vi "VisualizeRoomAlert.vi"() -> ()   [LabVIEW 2018, in "Visualization.lvlib" / "VisualizeSensor.lvclass"]
doc: "This VI listens for any measurement data associated with the provided PluginName and displays it to the user for analysis. The display is only suitable for data coming from the RoomAlert Plugin."
uses:
  VisualizeSensor.lvclass
  VisualizeBase/VisualizeBase_class/Requests/clUserEventType.ctl
  <vilib>/event_ctls.llb/usereventprio.ctl
  Sensor/SensorShared/clSensorData.ctl
  <vilib>/Utility/error.llb/Error Cluster From Error Code.vi
  <vilib>/ErrorRing/Error Ring.xnode
  <userlib>/NIST/NISTErrorLib/NISTErrorLib.lvlib
  VisualizeBase/VisualizeBase_class/VisualizeBase.lvclass
  Sensor/SensorShared/SensorShared.lvlib
  Sensor/SensorModule/SensorModule.lvlib
panel:
  out "LightTower":T1(array[cluster])
  out "String Results":string[](array[string])
  in  "Tab Control":enum32{"Chart"}(tab)
  out "Siemens":waveform(dbl)[](graph)=[{"t0"=timestamp(3657200531.6397257 s since 1904-01-01), "dt"=1.0, "Y"=[46.19]}, {"t0"=timestamp(3657200531.6397257 s since 1904-01-01), "dt"=1.0, "Y"=[2.0]}, {"t0"=timestamp(3657200531.6397257 s since 1904-01-01), "dt"=1.0, "Y"=[60.0]}]
  in  "PlotYAxis":u32[](array[numeric])=[0, 1, 0] max=1
  out "Incorrect DataType?":bool
  out "ErrorArray":errorcluster[](array[cluster])
  in  "PluginName":string="Sensor.RoomAlert0"
  in  "btnStop":bool
  in  "btnReset":bool
  in  "btnClear":bool
  # "0=Left Axis and 1=Right Axis"
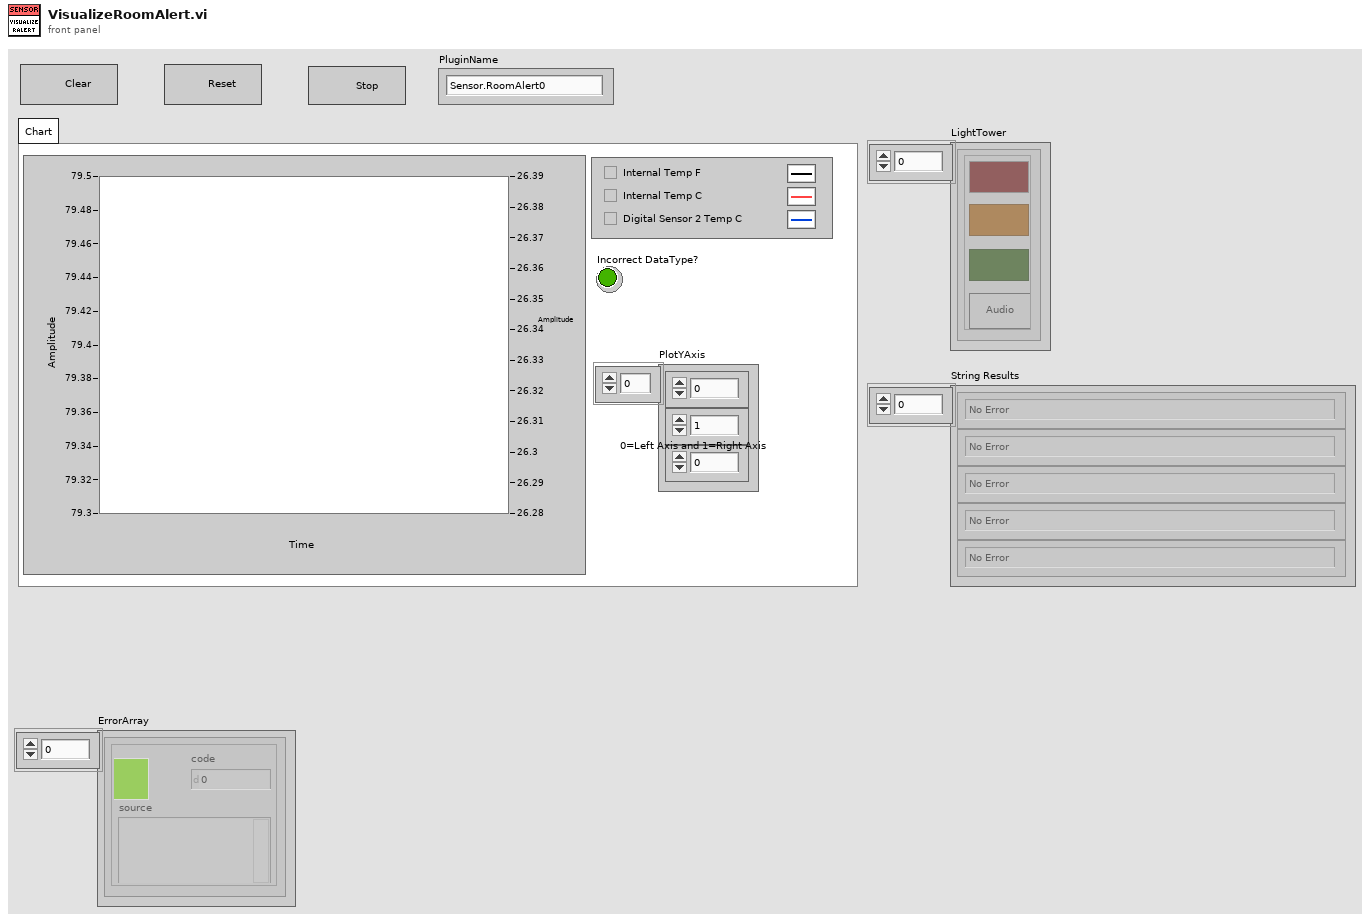
[diagram p1: front panel]
types:
  T1 = cluster{"Red":bool, "Amber":bool, "Green":bool, "Audio":bool}[]
  T2 = typedef "Visualization.lvlib/VisualizeBase.lvclass/clRequestEvents.ctl" = cluster{"StopRequest":refnum<user-event>, "ResetRequest":refnum<user-event>}
  T3 = typedef "SensorShared.lvlib/clBroadcastEvents.ctl" = cluster{"DidInit":refnum<user-event>, "StatusUpdate":refnum<user-event>, "ErrorReport":refnum<user-event>, "DidStop":refnum<user-event>, "PathToINI":refnum<user-event>, "SensorReport":refnum<user-event>, "SensorConfig":refnum<user-event>}
  T4 = typedef "SensorShared.lvlib/clSensorData.ctl" = cluster{"SensorType":string, "SensorData":variant}
  T5 = typedef "Visualization.lvlib/VisualizeBase.lvclass/clUserEventType.ctl" = cluster{"BusIndex":i8, "Data":variant}
  T6 = typedef "usereventprio.ctl" = enum32{"high priority", "normal priority"}
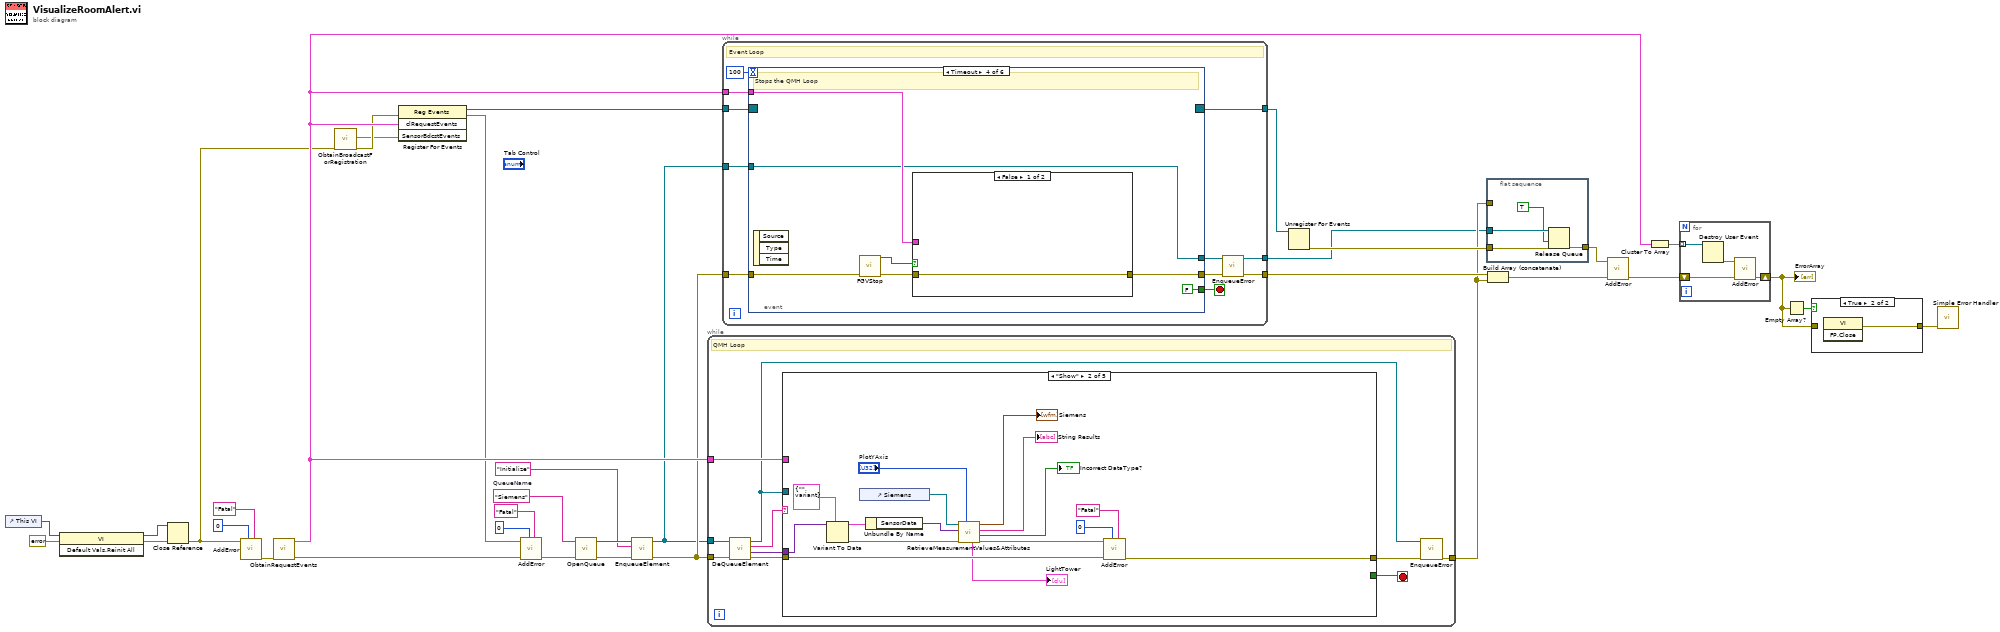
[diagram p0: block diagram]
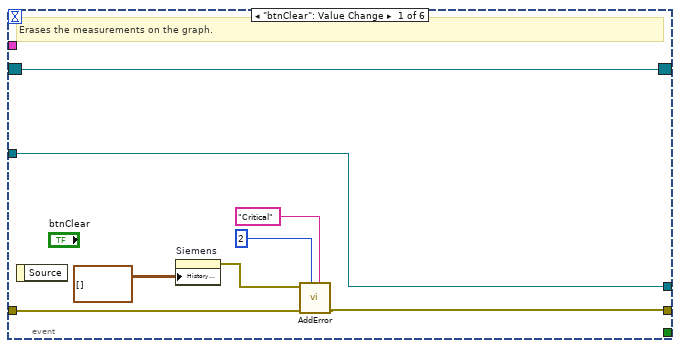
[diagram p2: hidden frame]
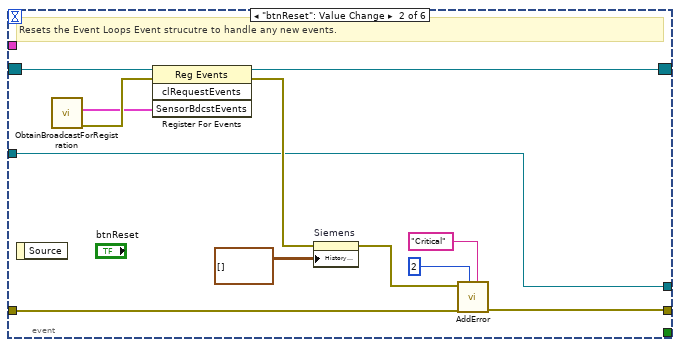
[diagram p3: hidden frame]
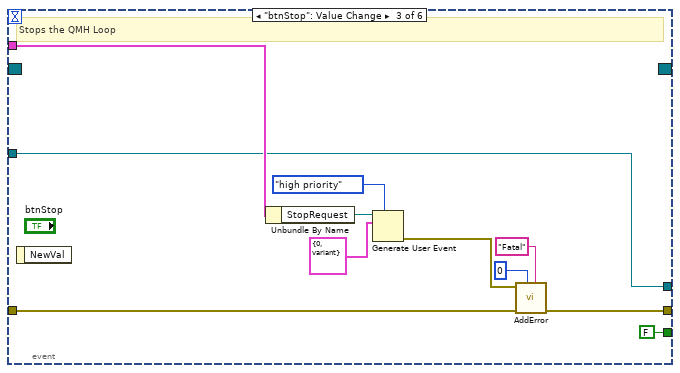
[diagram p4: hidden frame]
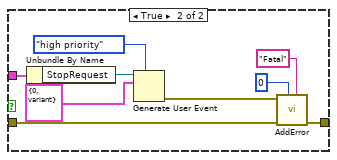
[diagram p5: hidden frame]
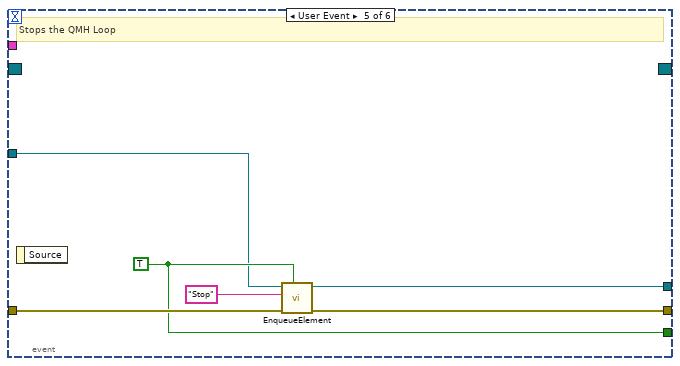
[diagram p6: hidden frame]
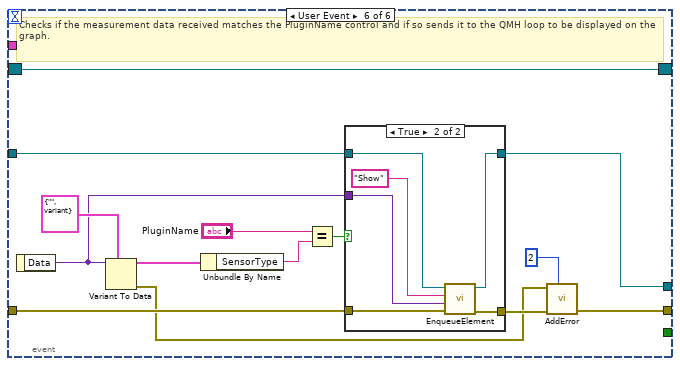
[diagram p7: hidden frame]
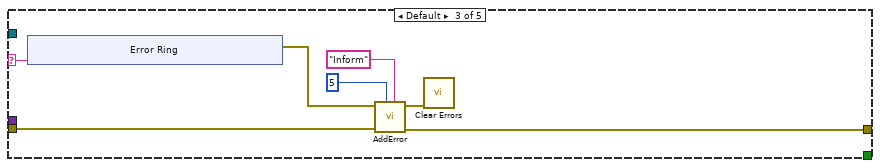
[diagram p10: hidden frame]
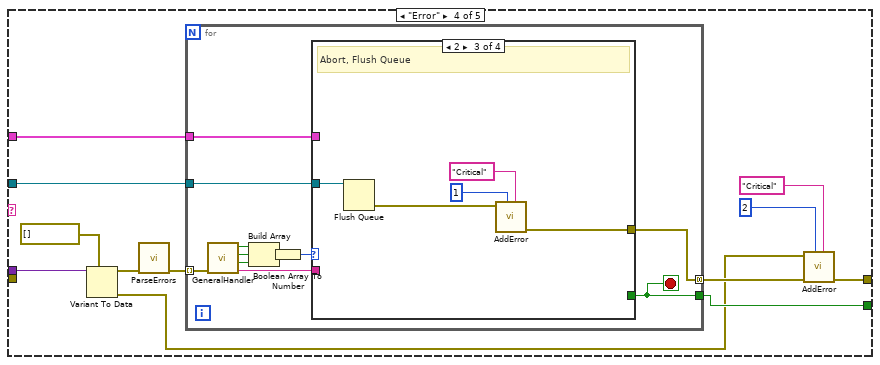
[diagram p11: hidden frame]
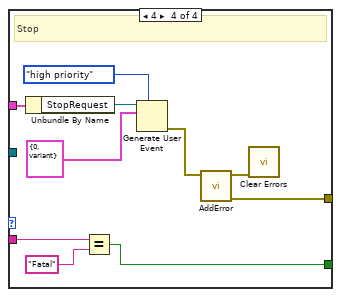
[diagram p14: hidden frame]
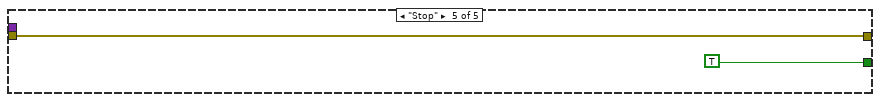
[diagram p15: hidden frame]
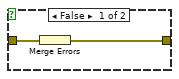
[diagram p16: hidden frame]
diagram:
  w10 = "Siemens"  # QueueName
  n1 = control-ref of="This VI"() -> (w24:refnum<vi>)
  n2 = invoke class="VI" method="Default Vals.Reinit All"(reference=w24, error in=errorcluster {"status"=FALSE, "code"=0, "source"=""} ("error in (no error)")) -> (reference out=w21:refnum<vi>, error out=w22:errorcluster)  [unwired: 1 in, 1 out]
  n3 = Close Reference(reference=w21, error in (no error)=w22) -> (error out=w12:errorcluster)
  n4 = call <userlib>:"AddError.vi"("Severity"="Fatal", "Priority"=u8 0, "error in (no error)"=w12) -> ("ErrorArray Out"=w34:errorcluster[])  [unwired: 7 in, 1 out]
  n5 = call "ObtainRequestEvents.vi"("Error"=w34) -> ("Error"=w19:errorcluster[], "clRequestEvents"=w26:T2)  [unwired: 9 in]
  n6 = call "ObtainBroadcastForRegistration.vi"("error in (no error)"=w12) -> ("error out"=w13:errorcluster, "SensorBdcstEvents"=w1:T3)  [unwired: 9 in]
  n7 = register-events(error in=w13, w26, w1) -> (reference out=w35:refnum<event-registration>, error out=w17:errorcluster)  [unwired: 1 in]
  n8 = call <userlib>:"AddError.vi"("Severity"="Fatal", "Priority"=u8 0, "ErrorArray In"=w19, "error in (no error)"=w17) -> ("ErrorArray Out"=w11:errorcluster[])  [unwired: 6 in, 1 out]
  n9 = call "OpenQueue.vi"("Error Array In"=w11, "QueueName"=w10) -> ("Error Array Out"=w8:errorcluster[], "queue out"=w9:refnum<queue>)  [unwired: 8 in]
  n10 = call "EnqueueElement.vi"("Error Array In"=w8, "Message"="Initialize", "queue in"=w9) -> ("Error Array Out"=w6:errorcluster[], "queue out"=w5:refnum<queue>)  [unwired: 7 in]
  n11 = while {
    tunnel: w6 -> [w39]
    tunnel: [w42] -> w14
    tunnel: w5 -> [w38]
    tunnel: w26 -> [w44]
    stop <- w45 stop-if-true
    # "QMH Loop"
    n12 = call "DeQueueElement.vi"("Error Array In"=w39, "Queue In"=w38) -> ("Error Array Out"=w37:errorcluster[], "Data"=w40:variant, "Message"=w41:string, "Queue Out"=w36:refnum<queue>)  [unwired: 6 in]
    n13 = case shown="\"Show\"" w41 {
      selector: w41 -> [_ _ w69 _ _]
      tunnel: w40 -> [_ w54 _ w88 _]
      tunnel: w37 -> [w46 w60 w67 _ w115]
      tunnel: [w46 w62 w66 w78 w115] -> w43
      tunnel: [_ _ _ w84 TRUE] -> w45
      tunnel: w44 -> [_ _ _ w83 _]
      tunnel: w36 -> [_ _ _ w82 _]
      frame "Initialize" {
      }
      frame "Show" {
        n14 = Variant To Data(type=T4 {"SensorType"="", "SensorData"=variant} ("clSensorData"), Variant=w54) -> (data=w52:T4, error out=w53:errorcluster)  [unwired: 1 in]
        n15 = control-ref of="Siemens"() -> (w61:refnum<vi>)
        n16 = Unbundle By Name(w52) -> ("SensorData"=w49:variant)
        n17 = call "RetrieveMeasurementValues&Attributes.vi"("PlotYScale"="PlotYAxis", "error in (no error)"=w53, "Variant"=w49, "WaveformChartReference"=w61) -> ("error out"=w56:errorcluster, "Incorrect DataType?"=→"Incorrect DataType?":bool, "Array Of Strings"=→"String Results":string[], "WaveformArrayOut"=→"Siemens":waveform(dbl)[], "LightTower"=→"LightTower":T1)  [unwired: 3 in]
        n18 = call <userlib>:"AddError.vi"("Severity"="Fatal" ("String"), "Priority"=u8 0, "ErrorArray In"=w60, "error in (no error)"=w56) -> ("ErrorArray Out"=w62:errorcluster[])  [unwired: 6 in, 1 out]
      }
      frame Default {
        n19 = xnode "Error Ring"("parameter 0"=w69) -> ("error out"=w68:errorcluster)
        n20 = call <userlib>:"AddError.vi"("Severity"="Inform" ("String"), "Priority"=u8 5, "ErrorArray In"=w67, "error in (no error)"=w68) -> ("ErrorArray Out"=w66:errorcluster[], "error out"=w65:errorcluster)  [unwired: 6 in]
        n21 = call <vilib>:"Clear Errors.vi"("error in (no error)"=w65) -> ()  [unwired: 5 in, 2 out]
      }
      frame "Error" {
        n22 = Variant To Data(type=errorcluster[] [], Variant=w88) -> (data=w86:errorcluster[], error out=w77:errorcluster)  [unwired: 1 in]
        n23 = call <userlib>:"ParseErrors.vi"("ErrorArray"=w86) -> ("ErrorArray"=w85:errorcluster[])  [unwired: 8 in, 2 out]
        n24 = for {
          tunnel: w85 -> [w99] mode=indexing
          tunnel: [w93] -> w79 mode=concatenating
          tunnel: [w91] -> w84
          tunnel: w83 -> [w90]
          tunnel: w82 -> [w89]
          stop <- w91 stop-if-true
          n25 = call <userlib>:"GeneralHandler.vi"("error in (no error)"=w99) -> ("Severity"=w92:string, "Stop"=w96:bool, "Abort"=w97:bool, "Continue"=w98:bool)  [unwired: 6 in, 1 out]
          n26 = Build Array(w98, w97, w96) -> (w95:bool[])
          n27 = Boolean Array To Number(Boolean array=w95) -> (number=w94:u32)
          n28 = case shown="2" w94 {
            tunnel: [_ _ w104 w113] -> w93
            tunnel: w92 -> [_ _ _ w106]
            tunnel: [_ _ _ w108] -> w91
            tunnel: w90 -> [_ _ _ w107]
            tunnel: w89 -> [_ _ w100 _]
            frame 0, Default {
              # "No Dialog"
            }
            frame 1 {
              # "Continue"
            }
            frame 2 {
              # "Abort, Flush Queue"
              n29 = Flush Queue(queue=w100) -> (error out=w103:errorcluster)  [unwired: 1 in, 2 out]
              n30 = call <userlib>:"AddError.vi"("Severity"="Critical" ("String"), "Priority"=u8 1, "error in (no error)"=w103) -> ("ErrorArray Out"=w104:errorcluster[])  [unwired: 7 in, 1 out]
            }
            frame 4 {
              # "Stop"
              n31 = Unbundle By Name(w107) -> ("StopRequest"=w114:refnum<user-event>)
              n32 = Equal?(x=w106, y="Fatal" ("x")) -> (x = y?=w108:bool)
              n33 = Generate User Event(priority (normal)=usereventprio."high priority", user event=w114, event data cluster=T5 {"BusIndex"=0, "Data"=variant} ("event data")) -> (error out=w112:errorcluster)  [unwired: 1 in, 1 out]
              n34 = call <userlib>:"AddError.vi"("error in (no error)"=w112) -> ("ErrorArray Out"=w113:errorcluster[], "error out"=w109:errorcluster)  [unwired: 9 in]
              n35 = call <vilib>:"Clear Errors.vi"("error in (no error)"=w109) -> ()  [unwired: 5 in, 2 out]
            }
          }
        }
        n36 = call <userlib>:"AddError.vi"("Severity"="Critical", "Priority"=u8 2, "ErrorArray In"=w79, "error in (no error)"=w77) -> ("ErrorArray Out"=w78:errorcluster[])  [unwired: 6 in, 1 out]
      }
      frame "Stop" {
      }
    }
    n37 = call "EnqueueError.vi"("Error Array In"=w43, "Queue in"=w36) -> ("Error Array Out"=w42:errorcluster[])  [unwired: 8 in, 1 out]
  }
  n38 = while {
    tunnel: w35 -> [w127]
    tunnel: [w121] -> w31
    tunnel: [w125] -> w33
    tunnel: w26 -> [w124]
    tunnel: w6 -> [w123]
    tunnel: w5 -> [w122]
    tunnel: [w118] -> w4
    stop <- w126 stop-if-true
    # "Event Loop"
    n39 = event shown="[3] Timeout" {
      selector: w127 -> [w129 w147 _ _ _ w190]
      dyn-events: [w129 w146 _ _ _ w190] -> w125
      timeout: 100 -> [_ _ _ _ _ _]
      tunnel: [_ _ FALSE ("Priority? (F)") FALSE ("Priority? (F)") w178 _] -> w126
      tunnel: [w132 w144 w151 w165 w180 w193] -> w120
      tunnel: w124 -> [_ _ w150 w164 _ _]
      tunnel: w123 -> [w133 w145 w158 w161 w181 w194]
      tunnel: w122 -> [w128 w137 w148 w162 w176 w195]
      tunnel: [w128 w137 w148 w162 w179 w191] -> w119
      event "btnClear": Value Change {
        # "Erases the measurements on the graph."
        n40 = event-data() -> ()  [unwired: 1 in, 1 out]
        n41 = property on="Siemens" class="WFChart (strict)"("History Data"=waveform(dbl)[][] []) -> (error out=w131:errorcluster)  [unwired: 2 in, 1 out]
        n42 = call <userlib>:"AddError.vi"("Severity"="Critical", "Priority"=u8 2, "ErrorArray In"=w133, "error in (no error)"=w131) -> ("ErrorArray Out"=w132:errorcluster[])  [unwired: 6 in, 1 out]
      }
      event "btnReset": Value Change {
        # "Resets the Event Loops Event strucutre to handle any new events."
        n43 = event-data() -> ()  [unwired: 1 in, 1 out]
        n44 = call "ObtainBroadcastForRegistration.vi"() -> ("error out"=w138:errorcluster, "SensorBdcstEvents"=w136:T3)  [unwired: 10 in]
        n45 = register-events(reference=w147, error in=w138, w136) -> (reference out=w146:refnum<event-registration>, error out=w140:errorcluster)  [unwired: 1 in]
        n46 = property on="Siemens" class="WFChart (strict)"(error in=w140, "History Data"=waveform(dbl)[][] []) -> (error out=w139:errorcluster)  [unwired: 1 in, 1 out]
        n47 = call <userlib>:"AddError.vi"("Severity"="Critical", "Priority"=u8 2, "ErrorArray In"=w145, "error in (no error)"=w139) -> ("ErrorArray Out"=w144:errorcluster[])  [unwired: 6 in, 1 out]
      }
      event "btnStop": Value Change {
        # "Stops the QMH Loop"
        n48 = event-data() -> ()  [unwired: 1 in, 1 out]
        n49 = Unbundle By Name(w150) -> ("StopRequest"=w156:refnum<user-event>)
        n50 = Generate User Event(priority (normal)=usereventprio."high priority", user event=w156, event data cluster=T5 {"BusIndex"=0, "Data"=variant} ("event data")) -> (error out=w157:errorcluster)  [unwired: 1 in, 1 out]
        n51 = call <userlib>:"AddError.vi"("Severity"="Fatal" ("String"), "Priority"=u8 0, "ErrorArray In"=w158, "error in (no error)"=w157) -> ("ErrorArray Out"=w151:errorcluster[])  [unwired: 6 in, 1 out]
      }
      event Timeout {
        # "Stops the QMH Loop"
        n52 = event-data() -> ()  [unwired: 1 in, 3 out]
        n53 = call "FGVStop.vi"("Error In"=w161) -> ("Error Out"=w159:errorcluster[], "Value"=w160:bool)  [unwired: 9 in]
        n54 = case shown="False" w160 {
          tunnel: w159 -> [w166 w175]
          tunnel: [w166 w168] -> w165
          tunnel: w164 -> [_ w167]
          frame False {
          }
          frame True {
            n55 = Unbundle By Name(w167) -> ("StopRequest"=w173:refnum<user-event>)
            n56 = Generate User Event(priority (normal)=usereventprio."high priority", user event=w173, event data cluster=T5 {"BusIndex"=0, "Data"=variant} ("event data")) -> (error out=w174:errorcluster)  [unwired: 1 in, 1 out]
            n57 = call <userlib>:"AddError.vi"("Severity"="Fatal" ("String"), "Priority"=u8 0, "ErrorArray In"=w175, "error in (no error)"=w174) -> ("ErrorArray Out"=w168:errorcluster[])  [unwired: 6 in, 1 out]
          }
        }
      }
      event User Event {
        w178 = TRUE ("Priority? (F)")
        # "Stops the QMH Loop"
        n58 = event-data() -> ()  [unwired: 1 in, 1 out]
        n59 = call "EnqueueElement.vi"("Priority? (F)"=w178, "Error Array In"=w181, "Message"="Stop", "queue in"=w176) -> ("Error Array Out"=w180:errorcluster[], "queue out"=w179:refnum<queue>)  [unwired: 6 in]
      }
      event User Event {
        # "Checks if the measurement data received matches the PluginName control and if so sends it to the QMH loop to be displayed on the graph."
        n60 = event-data() -> ("Data"=w187:variant)  [unwired: 1 in]
        n61 = Variant To Data(type=T4 {"SensorType"="", "SensorData"=variant} ("clSensorData"), Variant=w187) -> (data=w185:T4, error out=w186:errorcluster)  [unwired: 1 in]
        n62 = Unbundle By Name(w185) -> ("SensorType"=w184:string)
        n63 = Equal?(x="PluginName", y=w184) -> (x = y?=w182:bool)
        n64 = case shown="True" w182 {
          tunnel: [w196 w202] -> w192
          tunnel: w195 -> [w197 w201]
          tunnel: w194 -> [w196 w203]
          tunnel: [w197 w199] -> w191
          tunnel: w187 -> [_ w200]
          frame False {
          }
          frame True {
            n65 = call "EnqueueElement.vi"("Error Array In"=w203, "Data"=w200, "Message"="Show", "queue in"=w201) -> ("Error Array Out"=w202:errorcluster[], "queue out"=w199:refnum<queue>)  [unwired: 6 in]
          }
        }
        n66 = call <userlib>:"AddError.vi"("Priority"=u8 2, "ErrorArray In"=w192, "error in (no error)"=w186) -> ("ErrorArray Out"=w193:errorcluster[])  [unwired: 7 in, 1 out]
      }
    }
    n67 = call "EnqueueError.vi"("Error Array In"=w120, "Queue in"=w119) -> ("Error Array Out"=w121:errorcluster[], "Queue out"=w118:refnum<queue>)  [unwired: 8 in]
  }
  n68 = Unregister For Events(event registration refnum=w33) -> (error out=w30:errorcluster)  [unwired: 1 in]
  n69 = flat-sequence {
    tunnel: w30 -> [w207]
    tunnel: [w206] -> w28
    tunnel: w4 -> [w205]
    tunnel: w14 -> [_]
    frame #0 {
      n70 = Release Queue(queue=w205, force destroy? (F)=TRUE, error in (no error)=w207) -> (error out=w206:errorcluster)  [unwired: 2 out]
    }
  }
  n71 = Build Array (concatenate)(w31, w14) -> (w29:errorcluster[])
  n72 = call <userlib>:"AddError.vi"("ErrorArray In"=w29, "error in (no error)"=w28) -> ("ErrorArray Out"=w27:errorcluster[])  [unwired: 8 in, 1 out]
  n73 = Cluster To Array(cluster=w26) -> (array=w32:refnum<user-event>[])
  n74 = for {
    tunnel: w32 -> [w211] mode=indexing
    shift-right: [w210] -> w3
    shift-left: w27 -> [w209]
    n75 = Destroy User Event(user event=w211) -> (error out=w208:errorcluster)  [unwired: 1 in]
    n76 = call <userlib>:"AddError.vi"("ErrorArray In"=w209, "error in (no error)"=w208) -> ("ErrorArray Out"=w210:errorcluster[])  [unwired: 8 in, 1 out]
  }
  "ErrorArray" <- w3
  n77 = Empty Array?(array=w3) -> (empty?=w25:bool)
  n78 = case shown="True" w25 {
    tunnel: [w212 w214] -> w2
    tunnel: w3 -> [w213 _]
    frame False {
      n79 = Merge Errors(w213) -> (w212:errorcluster)
    }
    frame True {
      n80 = invoke class="VI" method="FP.Close"() -> (error out=w214:errorcluster)  [unwired: 3 in, 2 out]
    }
  }
  n81 = call <vilib>:"Simple Error Handler.vi"("error in (no error)"=w2) -> ()  [unwired: 4 in, 5 out]
